vi "Main.vi"() -> ()   [LabVIEW 2020]
panel:
  in  "OK Button":bool
  # "Is this VI running?"
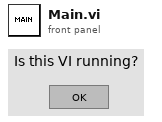
[diagram p1: front panel]
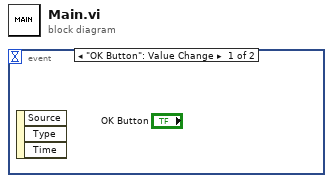
[diagram p0: block diagram]
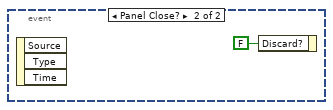
[diagram p2: hidden frame]
diagram:
  n1 = event shown="[0] \"OK Button\": Value Change" {
    selector: _ -> [_ _]
    dyn-events: _ -> [_ _]
    timeout: _ -> [_ _]
    event "OK Button": Value Change {
      n2 = event-data() -> ()  [unwired: 1 in, 3 out]
    }
    event Panel Close? {
      n3 = event-data() -> ()  [unwired: 1 in, 3 out]
      n4 = event-data("Discard?"=FALSE) -> ()  [unwired: 1 in, 1 out]
    }
  }
